vi "HFRR ADV v011 new software.vi"() -> ()   [LabVIEW 2025] (continued)
            n938 = local write "LIVE FEED MIN TEMP"(w1292) -> ()
            n939 = call "CAMERA LIVE FEED FGV.vi"("Enum - Menu"=CAMERA_LIVE_FEED_ENUM."CAMERA MINIMIZE") -> ()  [unwired: 9 in, 2 out]
          }
        }
        n940 = case shown="True" w1284 {
          selector: w1284 -> [_ w1290]
          frame False {
          }
          frame True {
            n941 = Not(x=w1290) -> (.not. x?=w1289:bool)
            n942 = local write "CAMERA ROI MIN TEMP"(w1289) -> ()
            n943 = call "IMAGE ANALYSIS.vi"("Enum"=POST_ANALYSIS_ENUM."MINIMIZE UI") -> ()  [unwired: 9 in, 2 out]
          }
        }
        n944 = local write "CAMERA ROI MAX TEMP"(TRUE ("CAMERA ROI MAX TEMP")) -> ()
      }
      frame "About" {
        n945 = local read "LIVE FEED MIN TEMP"() -> (w1296:bool)
        n946 = local write "LIVE FEED MAX TEMP"(TRUE ("LIVE FEED MAX TEMP")) -> ()
        n947 = local read "CAMERA ROI MIN TEMP"() -> (w1295:bool)
        n948 = case shown="True" w1296 {
          selector: w1296 -> [_ w1303]
          frame False {
          }
          frame True {
            n949 = Not(x=w1303) -> (.not. x?=w1302:bool)
            n950 = local write "LIVE FEED MIN TEMP"(w1302) -> ()
            n951 = call "CAMERA LIVE FEED FGV.vi"("Enum - Menu"=CAMERA_LIVE_FEED_ENUM."CAMERA MINIMIZE") -> ()  [unwired: 9 in, 2 out]
          }
        }
        n952 = case shown="True" w1295 {
          selector: w1295 -> [_ w1300]
          frame False {
          }
          frame True {
            n953 = Not(x=w1300) -> (.not. x?=w1299:bool)
            n954 = local write "CAMERA ROI MIN TEMP"(w1299) -> ()
            n955 = call "IMAGE ANALYSIS.vi"("Enum"=POST_ANALYSIS_ENUM."MINIMIZE UI") -> ()  [unwired: 9 in, 2 out]
          }
        }
        n956 = local write "CAMERA ROI MAX TEMP"(TRUE ("CAMERA ROI MIN TEMP")) -> ()
      }
      frame "Advance" {
        n957 = local read "LIVE FEED MIN TEMP"() -> (w1306:bool)
        n958 = local write "LIVE FEED MAX TEMP"(TRUE ("LIVE FEED MAX TEMP")) -> ()
        n959 = local read "CAMERA ROI MIN TEMP"() -> (w1304:bool)
        n960 = case shown="True" w1306 {
          selector: w1306 -> [_ w1313]
          frame False {
          }
          frame True {
            n961 = Not(x=w1313) -> (.not. x?=w1312:bool)
            n962 = local write "LIVE FEED MIN TEMP"(w1312) -> ()
            n963 = call "CAMERA LIVE FEED FGV.vi"("Enum - Menu"=CAMERA_LIVE_FEED_ENUM."CAMERA MINIMIZE") -> ()  [unwired: 9 in, 2 out]
          }
        }
        n964 = local write "CAMERA ROI MAX TEMP"(TRUE ("CAMERA ROI MAX TEMP")) -> ()
        n965 = case shown="True" w1304 {
          selector: w1304 -> [_ w1310]
          frame False {
          }
          frame True {
            n966 = Not(x=w1310) -> (.not. x?=w1309:bool)
            n967 = local write "CAMERA ROI MIN TEMP"(w1309) -> ()
            n968 = call "IMAGE ANALYSIS.vi"("Enum"=POST_ANALYSIS_ENUM."MINIMIZE UI") -> ()  [unwired: 9 in, 2 out]
          }
        }
      }
      frame "Mooha" {
        n969 = local read "LIVE FEED MIN TEMP"() -> (w1316:bool)
        n970 = local write "LIVE FEED MAX TEMP"(TRUE ("LIVE FEED MAX TEMP")) -> ()
        n971 = local read "CAMERA ROI MIN TEMP"() -> (w1314:bool)
        n972 = case shown="True" w1316 {
          selector: w1316 -> [_ w1323]
          frame False {
          }
          frame True {
            n973 = Not(x=w1323) -> (.not. x?=w1322:bool)
            n974 = local write "LIVE FEED MIN TEMP"(w1322) -> ()
            n975 = call "CAMERA LIVE FEED FGV.vi"("Enum - Menu"=CAMERA_LIVE_FEED_ENUM."CAMERA MINIMIZE") -> ()  [unwired: 9 in, 2 out]
          }
        }
        n976 = local write "CAMERA ROI MAX TEMP"(TRUE ("CAMERA ROI MAX TEMP")) -> ()
        n977 = case shown="True" w1314 {
          selector: w1314 -> [_ w1320]
          frame False {
          }
          frame True {
            n978 = Not(x=w1320) -> (.not. x?=w1319:bool)
            n979 = local write "CAMERA ROI MIN TEMP"(w1319) -> ()
            n980 = call "IMAGE ANALYSIS.vi"("Enum"=POST_ANALYSIS_ENUM."MINIMIZE UI") -> ()  [unwired: 9 in, 2 out]
          }
        }
      }
    }
    n981 = local read "Auto Start Test"() -> (w1060:bool)
    n982 = case shown="True" "sign in temp" {
      frame False {
      }
      frame True {
        w1096 = 1 ("y")
        n983 = local read "USERNAME"() -> (w1102:string)
        n984 = local read "USER ID"() -> (w1099:string)
        n985 = call <vilib>:"Trim Whitespace.vi"("string"=w1102) -> ("trimmed string"=w1101:string)  [unwired: 1 in]
        n986 = call <vilib>:"Trim Whitespace.vi"("string"=w1099) -> ("trimmed string"=w1100:string)  [unwired: 1 in]
        n987 = String Length(string=w1101) -> (length=w1098:i32)
        n988 = String Length(string=w1100) -> (length=w1097:i32)
        n989 = Greater?(x=w1098, y=w1096) -> (0:w1095:bool)
        n990 = Greater?(x=w1097, y=w1096) -> (0:w1094:bool)
        n991 = And(x=w1095, y=w1094) -> (x .and. y?=w1093:bool)
        n992 = case shown="True" w1093 {
          frame False {
            n993 = property on="Sign In" class="Bool (strict)"("DisabledEnum"=T17."Disabled" ("Disabled")) -> ()  [unwired: 2 in, 2 out]
          }
          frame True {
            n994 = property on="Sign In" class="Bool (strict)"("DisabledEnum"=T17."Enabled" ("Disabled")) -> ()  [unwired: 2 in, 2 out]
          }
        }
      }
    }
    n995 = local read "Air Temperature"() -> (w1077:bool)
    n996 = local read "Coefficient Of Friction"() -> (w1078:bool)
    n997 = case shown="False" w1060 {
      frame False {
        n998 = local read "Auto stop temp"() -> (w1090:bool)
        n999 = case shown="True" w1090 {
          frame False {
          }
          frame True {
            n1000 = local write "Auto Start Temp"(FALSE ("Auto Start Temp")) -> ()
          }
        }
      }
      frame True {
        "Auto stop temp" <- TRUE ("Auto stop temp")
      }
    }
    n1001 = local read "Humidity"() -> (w1076:bool)
    n1002 = case shown="\"HOME\"" w1087 {
      frame "HOME" {
        n1003 = local write "main tab sub"(enum32{"Page 1", "Page 2"}."Page 1" ("main tab sub")) -> ()
      }
      frame Default {
        n1004 = local write "main tab sub"(enum32{"Page 1", "Page 2"}."Page 2" ("main tab sub")) -> ()
      }
    }
    n1005 = case shown="True" w1086 {
      selector: w1086 -> [_ w1437]
      frame False {
      }
      frame True {
        n1006 = Not(x=w1437) -> (.not. x?=w1436:bool)
        n1007 = local write "Sign In"(w1436) -> ()
        n1008 = local write "Main Dashboard Buttons"(T23."Test Setup" ("Main Dashboard Buttons")) -> ()
      }
    }
    n1009 = case shown="\"Numeric Display\", Default" "Num/Graph" {
      frame "Numeric Display", Default {
        n1010 = property on="Single/Multiple" class="RadioBtnsControl (strict)"("Visible"=FALSE) -> ()  [unwired: 2 in, 2 out]
        n1011 = property on="Single - Graph" class="Ring (strict)"("Visible"=FALSE) -> ()  [unwired: 2 in, 2 out]
        n1012 = local write "Main Tab Display"(T4."Dashboard 1" ("Main Tab Display")) -> ()
      }
      frame "Graph Display" {
        n1013 = property on="Single/Multiple" class="RadioBtnsControl (strict)"("Visible"=TRUE) -> ()  [unwired: 2 in, 2 out]
        n1014 = case shown="\"Multiple\"" "Single/Multiple" {
          frame "Single ", Default {
            n1015 = property on="Single - Graph" class="Ring (strict)"("Visible"=TRUE) -> ()  [unwired: 2 in, 2 out]
            n1016 = local write "Main Tab Display"(T4."Dashboard 3" ("Main Tab Display")) -> ()
          }
          frame "Multiple" {
            n1017 = property on="Single - Graph" class="Ring (strict)"("Visible"=FALSE) -> ()  [unwired: 2 in, 2 out]
            n1018 = local write "Main Tab Display"(T4."Dashboard 2" ("Main Tab Display")) -> ()
          }
        }
      }
    }
    n1019 = local read "Stroke"() -> (w1075:bool)
    n1020 = local read "USERNAME"() -> (w1081:string)
    n1021 = local read "USER ID"() -> (w1080:string)
    n1022 = case shown="True" w1078 {
      selector: w1078 -> [_ w1363]
      frame False {
      }
      frame True {
        n1023 = Not(x=w1363) -> (.not. x?=w1362:bool)
        n1024 = local write "Coefficient Of Friction"(w1362) -> ()
        n1025 = local write "Tab Control 2"(T6."Coefficient Of Friction" ("Tab Control 2")) -> ()
      }
    }
    n1026 = case shown="True" w1077 {
      selector: w1077 -> [_ w1360]
      frame False {
      }
      frame True {
        n1027 = Not(x=w1360) -> (.not. x?=w1358:bool)
        n1028 = local write "Air Temperature"(w1358) -> ()
        n1029 = local write "Tab Control 2"(T6."Air Temperature" ("Tab Control 2")) -> ()
      }
    }
    n1030 = local write "Operator ID"(w1080) -> ()
    n1031 = case shown="True" w1075 {
      selector: w1075 -> [_ w1354]
      frame False {
      }
      frame True {
        n1032 = Not(x=w1354) -> (.not. x?=w1352:bool)
        n1033 = local write "Stroke"(w1352) -> ()
        n1034 = local write "Tab Control 2"(T6."Stroke" ("Tab Control 2")) -> ()
      }
    }
    n1035 = local write "tested by"(w1081) -> ()
    n1036 = case shown="True" w1076 {
      selector: w1076 -> [_ w1357]
      frame False {
      }
      frame True {
        n1037 = Not(x=w1357) -> (.not. x?=w1355:bool)
        n1038 = local write "Humidity"(w1355) -> ()
        n1039 = local write "Tab Control 2"(T6."Humidity" ("Tab Control 2")) -> ()
      }
    }
    n1040 = case shown="\"Calibration\"" "Main Dashboard Buttons" {
      tunnel: [T2."HOME" ("Main Tab") T2."Test Setup" ("Main Tab") T2."Acquire" ("Main Tab") T2."Adv Scar" ("Main Tab") T2."Adv Scar Report" ("Main Tab") T2."Compare Files" ("Main Tab") T2."Calibration" ("Main Tab") T2."About" ("Main Tab") T2."Advance" ("Main Tab")] -> w1059
      frame "Home", Default {
      }
      frame "Test Setup" {
      }
      frame "Dashboard" {
      }
      frame "Imaging" {
      }
      frame "Report" {
      }
      frame "Analysis" {
      }
      frame "Calibration" {
      }
      frame "About" {
      }
      frame "Advance" {
      }
    }
    n1041 = Wait (ms)(milliseconds to wait=u32 100) -> ()  [unwired: 1 out]
    n1042 = local read "Main Tab Display"() -> (w1079:T4)
    n1043 = local write "Main Tab"(w1059) -> ()
    n1044 = case shown="\"Dashboard 3\"" w1079 {
      frame "Dashboard 1", Default {
        n1045 = property on="Reset Graph" class="Bool (strict)"("Visible"=FALSE) -> ()  [unwired: 2 in, 2 out]
      }
      frame "Dashboard 2" {
        n1046 = property on="Reset Graph" class="Bool (strict)"("Visible"=TRUE) -> ()  [unwired: 2 in, 2 out]
      }
      frame "Dashboard 3" {
        n1047 = property on="Reset Graph" class="Bool (strict)"("Visible"=TRUE) -> ()  [unwired: 2 in, 2 out]
      }
    }
    n1048 = local read "SCAR MEASURMENT"() -> (w1067:enum32{"Auto Scar", "Manual Scar"})
    n1049 = local read "Humidity"() -> (w1082:bool)
    n1050 = local read "Cap Live Image"() -> (w1064:bool)
    n1051 = local read "Sample Temperature"() -> (w1074:bool)
    n1052 = local read "Air Temp vs Humidity"() -> (w1072:bool)
    n1053 = local read "Frequency"() -> (w1073:bool)
    n1054 = case shown="True" w1082 {
      frame False {
        n1055 = local write "Humidity On Command"(TRUE ("Humidity On Command")) -> ()
        n1056 = case shown="True" "Humidity Off Command" {
          selector: "Humidity Off Command" -> [_ w1370]
          frame False {
          }
          frame True {
            n1057 = stacked-sequence {
              frame #0 {
                n1058 = local read "WriteHumidity"() -> (w1372:string[])
                n1059 = Insert Into Array(array=w1372, new element="R;1" ("new element/subarray")) -> (w1373:string[])  [unwired: 1 in]
                n1060 = local write "WriteHumidity"(w1373) -> ()
              }
              frame #1 {
                n1061 = Wait (ms)(milliseconds to wait=u32 2000) -> ()  [unwired: 1 out]
              }
              frame #2 {
                n1062 = local read "EVENT LOG"() -> (w1379:string)
                n1063 = local read "WriteHumidity"() -> (w1376:string[])
                n1064 = call "Event Log.vi"("Content"="Humidity Control Off" ("string"), "EVENT LOG"=w1379) -> ("EVENT LOG"=w1380:string)  [unwired: 8 in, 1 out]
                n1065 = local write "EVENT LOG"(w1380) -> ()
                n1066 = Insert Into Array(array=w1376, new element="R;1" ("new element/subarray")) -> (w1377:string[])  [unwired: 1 in]
                n1067 = local write "WriteHumidity"(w1377) -> ()
              }
            }
            n1068 = Not(x=w1370) -> (.not. x?=w1369:bool)
            n1069 = local write "Humidity Off Command"(w1369) -> ()
          }
        }
      }
      frame True {
        n1070 = local write "Humidity Off Command"(TRUE ("Humidity Off Command")) -> ()
        n1071 = case shown="True" "Humidity On Command" {
          selector: "Humidity On Command" -> [_ w1384]
          frame False {
          }
          frame True {
            n1072 = stacked-sequence {
              frame #0 {
                n1073 = local read "Set Rh"() -> (w1390:dbl)
                n1074 = Number To Fractional String(number=w1390, precision (6)=i16 2) -> (F-format string=w1391:string)  [unwired: 2 in]
                n1075 = local read "WriteHumidity"() -> (w1388:string[])
                n1076 = Concatenate Strings("M;" ("new element/subarray"), w1391) -> (w1389:string)
                n1077 = Insert Into Array(array=w1388, new element=w1389) -> (w1387:string[])  [unwired: 1 in]
                n1078 = local write "WriteHumidity"(w1387) -> ()
              }
              frame #1 {
                n1079 = Wait (ms)(milliseconds to wait=u32 2000) -> ()  [unwired: 1 out]
              }
              frame #2 {
                n1080 = local read "Set Rh"() -> (w1398:dbl)
                n1081 = Number To Fractional String(number=w1398, precision (6)=i16 2) -> (F-format string=w1399:string)  [unwired: 2 in]
                n1082 = local read "WriteHumidity"() -> (w1396:string[])
                n1083 = Concatenate Strings("M;" ("new element/subarray"), w1399) -> (w1397:string)
                n1084 = Insert Into Array(array=w1396, new element=w1397) -> (w1395:string[])  [unwired: 1 in]
                n1085 = local write "WriteHumidity"(w1395) -> ()
              }
              frame #3 {
                n1086 = Wait (ms)(milliseconds to wait=u32 1500) -> ()  [unwired: 1 out]
              }
              frame #4 {
                (unwired) "% RH" ("string")
                (unwired) i16 2 ("precision (6)")
                (unwired) "M;" ("new element/subarray")
                n1087 = local read "Set Rh"() -> (w1406:dbl)
                n1088 = Number To Fractional String(number=w1406, precision (6)=i16 2) -> (F-format string=w1403:string)  [unwired: 2 in]
                n1089 = local read "WriteHumidity"() -> (w1408:string[])
                n1090 = Concatenate Strings("M;" ("new element/subarray"), w1403) -> (w1407:string)
                n1091 = Concatenate Strings("Humidity Set to : " ("string"), w1403, "% RH" ("string")) -> (w1401:string)
                n1092 = Insert Into Array(array=w1408, new element=w1407) -> (w1409:string[])  [unwired: 1 in]
                n1093 = disable-structure shown="Enabled" {
                  frame Enabled {
                    n1094 = local read "EVENT LOG"() -> (w1412:string)
                    n1095 = call "Event Log.vi"("Content"="Humidity Control On", "EVENT LOG"=w1412) -> ("EVENT LOG"=w1413:string)  [unwired: 8 in, 1 out]
                    n1096 = local write "EVENT LOG"(w1413) -> ()
                  }
                  frame Disabled {
                  }
                }
                n1097 = disable-structure shown="Enabled" {
                  disable-tunnel: w1401 -> [_ _]
                  frame Enabled {
                    n1098 = local read "EVENT LOG"() -> (w1415:string)
                    n1099 = call "Event Log.vi"("Content"="Humidity Control On", "EVENT LOG"=w1415) -> ("EVENT LOG"=w1416:string)  [unwired: 8 in, 1 out]
                    n1100 = local write "EVENT LOG"(w1416) -> ()
                  }
                  frame Disabled {
                  }
                }
                n1101 = local write "WriteHumidity"(w1409) -> ()
              }
            }
            n1102 = Not(x=w1384) -> (.not. x?=w1383:bool)
            n1103 = local write "Humidity On Command"(w1383) -> ()
          }
        }
      }
    }
    n1104 = Equal?(x=w1067, y=enum32{"Auto Scar", "Manual Scar"}."Auto Scar" ("SCAR MEASURMENT")) -> (x = y?=w1063:bool)
    n1105 = local read "TEST STANDARD"() -> (w1070:T3)
    n1106 = And(x=w1064, y=w1063) -> (x .and. y?=w1065:bool)
    n1107 = case shown="True" w1065 {
      selector: w1065 -> [_ w1169]
      tunnel: errorcluster {"status"=FALSE, "code"=0, "source"=""} ("error in (no error) 3") -> [_ w1170]
      frame False {
      }
      frame True {
        n1108 = stacked-sequence {
          tunnel: w1170 -> [_ _ _ _ _ _ _ w1218]
          tunnel: w1169 -> [_ _ _ _ _ w1199 _ _]
          frame #0 {
            n1109 = call "CAMERA LIVE FEED FGV.vi"("Enum - Menu"=CAMERA_LIVE_FEED_ENUM."CAMERA MINIMIZE") -> ()  [unwired: 9 in, 2 out]
          }
          frame #1 {
            n1110 = property on="Auto Scar Check  2" class="Clust (strict)"("Visible"=TRUE) -> ()  [unwired: 2 in, 2 out]
          }
          frame #2 {
            n1111 = String To Path(string="C:\\LAB-IQ\\Image Calibrate v01.dcf") -> (path=w1175:path)
            n1112 = Open/Create/Replace File ("Open File")(file path (use dialog)=w1175) -> (refnum out=w1176:refnum<file>)  [unwired: 5 in, 2 out]
            n1113 = for {
              N: 4 -> [_]
              tunnel: w1176 -> [w1182]
              i -> [w1178]
              n1114 = Read from Text File ("Read File")(file (use dialog)=w1182) -> (text=w1183:string)  [unwired: 3 in, 3 out]
              n1115 = String Subset(string=w1183, offset (0)=6, length (rest)=10 ("length (rest)")) -> (substring=w1179:string)
              n1116 = Fract/Exp String To Number(string=w1179) -> (number=w1177:dbl)  [unwired: 3 in, 1 out]
              n1117 = case shown="0" w1178 {
                tunnel: w1177 -> [w1184 w1185 _ w1186 _]
                frame 0 {
                  "5x Gain" <- w1184
                }
                frame 1 {
                  "10x Gain" <- w1185
                }
                frame 2 {
                }
                frame 3 {
                  "100x gain" <- w1186
                }
                frame 4, Default {
                }
              }
            }
          }
          frame #3 {
            n1118 = local read "FILE 3"() -> (w1192:string)
            n1119 = call <vilib>:"Trim Whitespace.vi"("string"="C:\\LAB-IQ\\images\\") -> ("trimmed string"=w1194:string)  [unwired: 1 in]
            n1120 = String To Path(string=w1194) -> (path=w1193:path)
            n1121 = Concatenate Strings(w1192, ".png" ("string")) -> (w1191:string)
            n1122 = Build Path(base path=w1193, name or relative path=w1191) -> (appended path=w1189:path)
            "Image path" <- w1189
            n1123 = Path To String(path=w1189) -> (string=w1188:string)
            n1124 = call "CAMERA LIVE FEED FGV.vi"("Enum - Menu"=CAMERA_LIVE_FEED_ENUM."CAMERA SAVE", "Image Path"=w1188) -> ()  [unwired: 8 in, 2 out]
          }
          frame #4 {
            n1125 = One Button Dialog(message="Image saved successfully") -> ()  [unwired: 1 in, 1 out]
          }
          frame #5 {
            n1126 = local read "TEST STANDARD"() -> (w1198:T3)
            n1127 = local read "Magnification len live scar"() -> (w1210:string)
            n1128 = Not(x=w1199) -> (.not. x?=w1200:bool)
            n1129 = local write "Cap Live Image"(w1200) -> ()
            n1130 = case shown="\"ISO 12156\"" w1198 {
              tunnel: ["ASTM D6079" "ISO 12156"] -> w1197
              frame "ASTM D6079", Default {
              }
              frame "ISO 12156" {
              }
            }
            n1131 = case shown="\"5x\", Default" w1210 {
              tunnel: [w1213 w1214] -> w1209
              frame "5x", Default {
                n1132 = local read "5x Gain"() -> (w1213:dbl)
              }
              frame "10x" {
                # "5x"
                n1133 = local read "10x Gain"() -> (w1214:dbl)
              }
            }
            n1134 = local read "Image path"() -> (w1208:path)
            n1135 = local read "FILE 3"() -> (w1201:string)
            n1136 = call "EDGE DETCTION.vi"("GAIN VALUE"=w1209, "Image Path"=w1208) -> ("error out"=w1207:errorcluster, "return value"=w1206:cluster{string, string, dbl, dbl, dbl})  [unwired: 8 in]
            n1137 = Bundle By Name(cluster=T24 {"File Name"="", "Test Method"="", "Operator"="", "Fuel Description"="", "Date and time"=""} ("Main Ref"), "File Name"=w1201, "Test Method"=w1197) -> (w1202:T24)
            n1138 = call "duf file read.vi"("error in (no error)"=w1207, "Main Ref"=w1202) -> ("error out"=w1205:errorcluster, "Main Ref 2"=w1203:T24)  [unwired: 8 in]
            n1139 = call "EDGE DETECTION REPORT.vi"("error in (no error)"=w1205, "return value 2"=w1206, "Main Ref"=w1203) -> ()  [unwired: 8 in, 1 out]
          }
          frame #6 {
            n1140 = property on="Auto Scar Check  2" class="Clust (strict)"("Visible"=FALSE) -> ()  [unwired: 2 in, 2 out]
          }
          frame #7 {
            n1141 = call "CAMERA LIVE FEED FGV.vi"("Enum - Menu"=CAMERA_LIVE_FEED_ENUM."CAMERA MINIMIZE", "error in (no error)"=w1218) -> ()  [unwired: 8 in, 2 out]
            n1142 = local write "Main Dashboard Buttons"(T1."Home" ("Main Dashboard Buttons")) -> ()
            n1143 = local write "Main Tab"(T2."HOME" ("Main Tab")) -> ()
          }
        }
      }
    }
    n1144 = local read "Heater Button"() -> (w1071:bool)
    n1145 = case shown="True" w1073 {
      selector: w1073 -> [_ w1348]
      frame False {
      }
      frame True {
        n1146 = Not(x=w1348) -> (.not. x?=w1346:bool)
        n1147 = local write "Frequency"(w1346) -> ()
        n1148 = local write "Tab Control 2"(T6."Frequency" ("Tab Control 2")) -> ()
      }
    }
    n1149 = case shown="True" w1072 {
      selector: w1072 -> [_ w1345]
      frame False {
      }
      frame True {
        n1150 = Not(x=w1345) -> (.not. x?=w1343:bool)
        n1151 = local write "Air Temp vs Humidity"(w1343) -> ()
        n1152 = local write "Tab Control 2"(T6."Air Temp vs Rh" ("Tab Control 2")) -> ()
      }
    }
    n1153 = case shown="True" w1074 {
      selector: w1074 -> [_ w1351]
      frame False {
      }
      frame True {
        n1154 = Not(x=w1351) -> (.not. x?=w1349:bool)
        n1155 = local write "Sample Temperature"(w1349) -> ()
        n1156 = local write "Tab Control 2"(T6."Sample Temperature" ("Tab Control 2")) -> ()
      }
    }
    n1157 = case shown="\"Custom\"" w1070 {
      frame "ASTM D6079", Default {
        w1324 = "ASTM D6079 TEST CONDITIONS" ("Standard 2")
        n1158 = local write "Standard 2"(w1324) -> ()
        n1159 = local write "Standard"(w1324) -> ()
      }
      frame "ISO 12156" {
        w1325 = "ISO 12156 TEST CONDITIONS" ("Standard 2")
        n1160 = local write "Standard 2"(w1325) -> ()
        n1161 = local write "Standard"(w1325) -> ()
      }
      frame "CEC F-096-A-06" {
        w1326 = "CEC F-096-A-06 TEST CONDITIONS" ("Standard 2")
        n1162 = local write "Standard 2"(w1326) -> ()
        n1163 = local write "Standard"(w1326) -> ()
      }
      frame "Custom" {
        w1327 = "CUSTOM TEST CONDITIONS" ("Standard 2")
        n1164 = local write "Standard 2"(w1327) -> ()
        n1165 = local write "Standard"(w1327) -> ()
      }
    }
    n1166 = case shown="True" w1071 {
      frame False {
        n1167 = local write "Temperature On Command"(TRUE ("Temperature On Command")) -> ()
        n1168 = case shown="True" "Temperature Off Command" {
          selector: "Temperature Off Command" -> [_ w1331]
          frame False {
          }
          frame True {
            n1169 = Not(x=w1331) -> (.not. x?=w1330:bool)
            n1170 = local read "EVENT LOG"() -> (w1334:string)
            n1171 = local write "Temperature Off Command"(w1330) -> ()
            n1172 = call "Event Log.vi"("Content"="Heater Off", "EVENT LOG"=w1334) -> ("EVENT LOG"=w1333:string)  [unwired: 8 in, 1 out]
            n1173 = local write "EVENT LOG"(w1333) -> ()
          }
        }
      }
      frame True {
        n1174 = local write "Temperature Off Command"(TRUE ("Temperature Off Command")) -> ()
        n1175 = case shown="True" "Temperature On Command" {
          selector: "Temperature On Command" -> [_ w1338]
          frame False {
          }
          frame True {
            n1176 = Not(x=w1338) -> (.not. x?=w1337:bool)
            n1177 = local write "Temperature On Command"(w1337) -> ()
            n1178 = disable-structure shown="Enabled" {
              disable-tunnel: "Heater On" -> [w1340 _]
              frame Enabled {
                n1179 = local read "EVENT LOG"() -> (w1341:string)
                n1180 = call "Event Log.vi"("Content"=w1340, "EVENT LOG"=w1341) -> ("EVENT LOG"=w1342:string)  [unwired: 8 in, 1 out]
                n1181 = local write "EVENT LOG"(w1342) -> ()
              }
              frame Disabled {
              }
            }
          }
        }
      }
    }
    n1182 = local read "Main Tab"() -> (w1062:T2)
    n1183 = case shown="\"About\"" w1062 {
      frame "HOME", Default {
        w1105 = T17."Enabled" ("Disabled")
        n1184 = local read "Service Password enable"() -> (w1107:bool)
        n1185 = property on="Imaging" class="Bool (strict)"("DisabledEnum"=w1105) -> ()  [unwired: 2 in, 2 out]
        n1186 = property on="Dashboard" class="Bool (strict)"("DisabledEnum"=w1105) -> ()  [unwired: 2 in, 2 out]
        n1187 = property on="Test Setup" class="Bool (strict)"("DisabledEnum"=w1105) -> ()  [unwired: 2 in, 2 out]
        n1188 = property on="Analysis" class="Bool (strict)"("DisabledEnum"=w1105) -> ()  [unwired: 2 in, 2 out]
        n1189 = property on="Home" class="Bool (strict)"("DisabledEnum"=w1105) -> ()  [unwired: 2 in, 2 out]
        n1190 = property on="Report" class="Bool (strict)"("DisabledEnum"=w1105) -> ()  [unwired: 2 in, 2 out]
        n1191 = property on="Main Dashboard Buttons" class="RadioBtnsControl (strict)"("DisabledEnum"=w1105) -> ()  [unwired: 2 in, 2 out]
        n1192 = property on="Calibration" class="Bool (strict)"("DisabledEnum"=w1105) -> ()  [unwired: 2 in, 2 out]
        n1193 = case shown="True" w1107 {
          tunnel: [T17."Disabled" ("Disabled") T17."Enabled" ("Disabled")] -> w1106
          frame False {
          }
          frame True {
          }
        }
        n1194 = property on="About" class="Bool (strict)"("DisabledEnum"=w1106) -> ()  [unwired: 2 in, 2 out]
      }
      frame "Test Setup" {
        w1112 = T17."Enabled" ("Disabled")
        n1195 = local read "Service Password enable"() -> (w1111:bool)
        n1196 = property on="Dashboard" class="Bool (strict)"("DisabledEnum"=T17."Disabled" ("Disabled")) -> ()  [unwired: 2 in, 2 out]
        n1197 = property on="Imaging" class="Bool (strict)"("DisabledEnum"=w1112) -> ()  [unwired: 2 in, 2 out]
        n1198 = property on="Analysis" class="Bool (strict)"("DisabledEnum"=w1112) -> ()  [unwired: 2 in, 2 out]
        n1199 = property on="Home" class="Bool (strict)"("DisabledEnum"=w1112) -> ()  [unwired: 2 in, 2 out]
        n1200 = property on="Report" class="Bool (strict)"("DisabledEnum"=w1112) -> ()  [unwired: 2 in, 2 out]
        n1201 = property on="Test Setup" class="Bool (strict)"("DisabledEnum"=w1112) -> ()  [unwired: 2 in, 2 out]
        n1202 = case shown="True" w1111 {
          tunnel: [T17."Disabled" ("Disabled") T17."Enabled" ("Disabled")] -> w1110
          frame False {
          }
          frame True {
          }
        }
        n1203 = property on="About" class="Bool (strict)"("DisabledEnum"=w1110) -> ()  [unwired: 2 in, 2 out]
      }
      frame "Adv Scar" {
        w1119 = T17."Enabled" ("Disabled")
        n1204 = property on="Dashboard" class="Bool (strict)"("DisabledEnum"=T17."Disabled" ("Disabled")) -> ()  [unwired: 2 in, 2 out]
        n1205 = property on="Imaging" class="Bool (strict)"("DisabledEnum"=w1119) -> ()  [unwired: 2 in, 2 out]
        n1206 = property on="Analysis" class="Bool (strict)"("DisabledEnum"=w1119) -> ()  [unwired: 2 in, 2 out]
        n1207 = property on="Home" class="Bool (strict)"("DisabledEnum"=w1119) -> ()  [unwired: 2 in, 2 out]
        n1208 = property on="Report" class="Bool (strict)"("DisabledEnum"=w1119) -> ()  [unwired: 2 in, 2 out]
        n1209 = property on="Test Setup" class="Bool (strict)"("DisabledEnum"=w1119) -> ()  [unwired: 2 in, 2 out]
        n1210 = local read "Service Password enable"() -> (w1117:bool)
        n1211 = case shown="True" w1117 {
          tunnel: [T17."Disabled" ("Disabled") T17."Enabled" ("Disabled")] -> w1116
          frame False {
          }
          frame True {
          }
        }
        n1212 = property on="About" class="Bool (strict)"("DisabledEnum"=w1116) -> ()  [unwired: 2 in, 2 out]
      }
      frame "Calibration" {
        w1122 = T17."Enabled" ("Disabled")
        n1213 = property on="Dashboard" class="Bool (strict)"("DisabledEnum"=T17."Disabled" ("Disabled")) -> ()  [unwired: 2 in, 2 out]
        n1214 = property on="Imaging" class="Bool (strict)"("DisabledEnum"=w1122) -> ()  [unwired: 2 in, 2 out]
        n1215 = property on="Analysis" class="Bool (strict)"("DisabledEnum"=w1122) -> ()  [unwired: 2 in, 2 out]
        n1216 = property on="Home" class="Bool (strict)"("DisabledEnum"=w1122) -> ()  [unwired: 2 in, 2 out]
        n1217 = property on="Report" class="Bool (strict)"("DisabledEnum"=w1122) -> ()  [unwired: 2 in, 2 out]
        n1218 = property on="Test Setup" class="Bool (strict)"("DisabledEnum"=w1122) -> ()  [unwired: 2 in, 2 out]
        n1219 = local read "Service Password enable"() -> (w1124:bool)
        n1220 = property on="Calibration" class="Bool (strict)"("DisabledEnum"=w1122) -> ()  [unwired: 2 in, 2 out]
        n1221 = case shown="True" w1124 {
          tunnel: [T17."Disabled" ("Disabled") T17."Enabled" ("Disabled")] -> w1123
          frame False {
          }
          frame True {
          }
        }
        n1222 = property on="About" class="Bool (strict)"("DisabledEnum"=w1123) -> ()  [unwired: 2 in, 2 out]
      }
      frame "Adv Scar Report" {
        w1130 = T17."Enabled" ("Disabled")
        n1223 = property on="Dashboard" class="Bool (strict)"("DisabledEnum"=T17."Disabled" ("Disabled")) -> ()  [unwired: 2 in, 2 out]
        n1224 = property on="Imaging" class="Bool (strict)"("DisabledEnum"=w1130) -> ()  [unwired: 2 in, 2 out]
        n1225 = property on="Analysis" class="Bool (strict)"("DisabledEnum"=w1130) -> ()  [unwired: 2 in, 2 out]
        n1226 = property on="Home" class="Bool (strict)"("DisabledEnum"=w1130) -> ()  [unwired: 2 in, 2 out]
        n1227 = property on="Report" class="Bool (strict)"("DisabledEnum"=w1130) -> ()  [unwired: 2 in, 2 out]
        n1228 = property on="Test Setup" class="Bool (strict)"("DisabledEnum"=w1130) -> ()  [unwired: 2 in, 2 out]
        n1229 = local read "Service Password enable"() -> (w1129:bool)
        n1230 = case shown="True" w1129 {
          tunnel: [T17."Disabled" ("Disabled") T17."Enabled" ("Disabled")] -> w1128
          frame False {
          }
          frame True {
          }
        }
        n1231 = property on="About" class="Bool (strict)"("DisabledEnum"=w1128) -> ()  [unwired: 2 in, 2 out]
      }
      frame "Compare Files" {
        w1136 = T17."Enabled" ("Disabled")
        n1232 = local read "Service Password enable"() -> (w1135:bool)
        n1233 = property on="Dashboard" class="Bool (strict)"("DisabledEnum"=T17."Disabled" ("Disabled")) -> ()  [unwired: 2 in, 2 out]
        n1234 = property on="Imaging" class="Bool (strict)"("DisabledEnum"=w1136) -> ()  [unwired: 2 in, 2 out]
        n1235 = property on="Analysis" class="Bool (strict)"("DisabledEnum"=w1136) -> ()  [unwired: 2 in, 2 out]
        n1236 = property on="Home" class="Bool (strict)"("DisabledEnum"=w1136) -> ()  [unwired: 2 in, 2 out]
        n1237 = property on="Report" class="Bool (strict)"("DisabledEnum"=w1136) -> ()  [unwired: 2 in, 2 out]
        n1238 = property on="Test Setup" class="Bool (strict)"("DisabledEnum"=w1136) -> ()  [unwired: 2 in, 2 out]
        n1239 = case shown="True" w1135 {
          tunnel: [T17."Disabled" ("Disabled") T17."Enabled" ("Disabled")] -> w1134
          frame False {
          }
          frame True {
          }
        }
        n1240 = property on="About" class="Bool (strict)"("DisabledEnum"=w1134) -> ()  [unwired: 2 in, 2 out]
      }
      frame "Acquire" {
        n1241 = local read "Service Password enable"() -> (w1141:bool)
        n1242 = property on="Test Setup" class="Bool (strict)"("DisabledEnum"=T17."Disabled" ("Disabled")) -> ()  [unwired: 2 in, 2 out]
        n1243 = local read "Auto Start Test"() -> (w1143:bool)
        n1244 = local read "RUN"() -> (w1145:bool)
        n1245 = case shown="True" w1141 {
          tunnel: [T17."Disabled" ("Disabled") T17."Enabled" ("Disabled")] -> w1142
          frame False {
          }
          frame True {
          }
        }
        n1246 = Or(x=w1145, y=w1143) -> (x .or. y?=w1144:bool)
        n1247 = case shown="True" w1144 {
          tunnel: [T17."Enabled" ("Disabled") T17."Disabled" ("Disabled")] -> w1140
          frame False {
          }
          frame True {
          }
        }
        n1248 = property on="About" class="Bool (strict)"("DisabledEnum"=w1142) -> ()  [unwired: 2 in, 2 out]
        n1249 = property on="Imaging" class="Bool (strict)"("DisabledEnum"=w1140) -> ()  [unwired: 2 in, 2 out]
        n1250 = property on="Dashboard" class="Bool (strict)"("DisabledEnum"=w1140) -> ()  [unwired: 2 in, 2 out]
        n1251 = property on="Analysis" class="Bool (strict)"("DisabledEnum"=w1140) -> ()  [unwired: 2 in, 2 out]
        n1252 = property on="Home" class="Bool (strict)"("DisabledEnum"=w1140) -> ()  [unwired: 2 in, 2 out]
        n1253 = property on="Report" class="Bool (strict)"("DisabledEnum"=w1140) -> ()  [unwired: 2 in, 2 out]
        n1254 = property on="Calibration" class="Bool (strict)"("DisabledEnum"=w1140) -> ()  [unwired: 2 in, 2 out]
      }
      frame "About" {
        n1255 = local read "FILE"() -> (w1159:string)
        n1256 = local read "TEST FILE NAM,E SAVED"() -> (w1152:bool)
        n1257 = call <vilib>:"Trim Whitespace.vi"("string"=w1159) -> ("trimmed string"=w1158:string)  [unwired: 1 in]
        n1258 = local read "Auto Start Test"() -> (w1162:bool)
        n1259 = String Length(string=w1158) -> (length=w1157:i32)
        n1260 = Greater?(x=w1157, y=1) -> (0:w1154:bool)
        n1261 = And(x=w1154, y=w1152) -> (x .and. y?=w1153:bool)
        n1262 = local read "RUN"() -> (w1164:bool)
        n1263 = case shown="True" w1153 {
          tunnel: [T17."Disabled" ("Disabled") T17."Enabled" ("Disabled")] -> w1155
          frame False {
          }
          frame True {
          }
        }
        n1264 = Or(x=w1164, y=w1162) -> (x .or. y?=w1163:bool)
        n1265 = property on="About" class="Bool (strict)"("DisabledEnum"=T17."Enabled" ("Disabled")) -> ()  [unwired: 2 in, 2 out]
        n1266 = case shown="False" w1163 {
          tunnel: [T17."Enabled" ("Disabled") T17."Disabled" ("Disabled")] -> w1161
          frame False {
          }
          frame True {
          }
        }
        n1267 = property on="Dashboard" class="Bool (strict)"("DisabledEnum"=w1155) -> ()  [unwired: 2 in, 2 out]
        n1268 = property on="Test Setup" class="Bool (strict)"("DisabledEnum"=T17."Disabled" ("Disabled")) -> ()  [unwired: 2 in, 2 out]
        n1269 = property on="Imaging" class="Bool (strict)"("DisabledEnum"=w1161) -> ()  [unwired: 2 in, 2 out]
        n1270 = property on="Analysis" class="Bool (strict)"("DisabledEnum"=w1161) -> ()  [unwired: 2 in, 2 out]
        n1271 = property on="Home" class="Bool (strict)"("DisabledEnum"=w1161) -> ()  [unwired: 2 in, 2 out]
        n1272 = property on="Report" class="Bool (strict)"("DisabledEnum"=w1161) -> ()  [unwired: 2 in, 2 out]
      }
    }
    n1273 = local read "Quit"() -> (w1089:bool)
    "Single" <- "Single - Graph"
  }
  n1274 = disable-structure shown="Disabled" {
    disable-tunnel: [w1441 _] -> w39
    disable-tunnel: _ -> [w1440 _]
    frame Disabled {
      n1275 = while {
        tunnel: w1440 -> [_]
        tunnel: [w1442] -> w1441
        tunnel: [w1443] -> _
        i -> [w1443]
        stop <- w1442 stop-if-true
        w1459 = u16 10 items=["1.0"=10, "1.5"=15, "2.0"=20] ("stop bits (10: 1 bit)")
        n1276 = Wait (ms)(milliseconds to wait=u32 10) -> ()  [unwired: 1 out]
        n1277 = call-poly "VISA Configure Serial Port"("VISA resource name"=refnum<visa-resource-name> "ASRL1::INSTR" ("COM PORT"), "timeout (10sec)"=u32 10, "baud rate (9600)"=u32 57600, "data bits (8)"=u16 8, "stop bits (10: 1 bit)"=w1459) -> ("VISA resource name out"=w1445:refnum<visa-resource-name>, "error out"=w1454:errorcluster)  [unwired: 9 in]
        n1278 = VISA Read(VISA resource name=w1445, byte count=u32 2 ("byte count (0)")) -> (read buffer=w1453:string)  [unwired: 1 in, 3 out]
        n1279 = String Subset(string=w1453, offset (0)=0, length (rest)=2 ("length (rest)")) -> (substring=w1452:string)
        n1280 = Match Pattern(string=w1452, regular expression="<>") -> (offset past match=w1449:i32)  [unwired: 1 in, 3 out]
        n1281 = Greater Or Equal?(x=w1449, y=0) -> (x >= y?=w1444:bool)
        n1282 = case shown="True" w1444 {
          tunnel: w1445 -> [_ w1463]
          tunnel: w1454 -> [_ w1462]
          frame False {
          }
          frame True {
            n1283 = VISA Read(VISA resource name=w1463, byte count=u32 32 ("byte count (0)"), error in (no error)=w1462) -> (read buffer=w1461:string)  [unwired: 3 out]
            n1284 = String Subset(string=w1461, offset (0)=0, length (rest)=8 ("length (rest)")) -> (substring=w1465:string)
            n1285 = String Subset(string=w1461, offset (0)=8, length (rest)=8 ("length (rest)")) -> (substring=w1466:string)
            n1286 = Decimal String To Number(string=w1466) -> (number=w1473:i32)  [unwired: 2 in, 1 out]
            n1287 = Decimal String To Number(string=w1465) -> (number=w1469:i32)  [unwired: 2 in, 1 out]
            n1288 = Divide(x=w1473, y=10000) -> ()  [unwired: 1 out]
            n1289 = Divide(x=w1469, y=1000000) -> ()  [unwired: 1 out]
          }
        }
        n1290 = local read "Quit"() -> (w1442:bool)
      }
    }
    frame Enabled {
    }
  }
  n1291 = while {
    shift-right: [w1488] -> w52
    shift-left: _ -> [w1479]
    shift-right: [w1487] -> w51
    shift-left: errorcluster {"status"=TRUE, "code"=0, "source"="Init"} ("error IO") -> [w1481]
    tunnel: [w1476] -> w42
    tunnel: [w1486] -> _
    i -> [w1486]
    stop <- w1476 stop-if-true
    n1292 = local read "Port 1a"() -> (w1482:bool)
    n1293 = local read "Port 3"() -> (w1483:bool)
    n1294 = local read "Com Port 1"() -> (w1480:refnum<visa-resource-name>)
    n1295 = Or(x=w1483, y=w1482) -> (x .or. y?=w1485:bool)
    n1296 = Unbundle(w1481) -> ("status"=→"Port 3":bool)  [unwired: 2 out]
    n1297 = Not Equal?(x=w1480, y=w1479) -> (x != y?=w1477:bool)
    n1298 = case shown="True" w1485 {
      frame False {
        w1491 = TRUE ("Visible")
        n1299 = property on="Port 1a" class="Bool (strict)"("Visible"=w1491) -> ()  [unwired: 2 in, 2 out]
        n1300 = property on="Port 3" class="Bool (strict)"("Visible"=w1491) -> ()  [unwired: 2 in, 2 out]
      }
      frame True {
        w1492 = TRUE ("Visible")
        n1301 = property on="Port 1a" class="Bool (strict)"("Visible"=w1492) -> ()  [unwired: 2 in, 2 out]
        n1302 = property on="Port 3" class="Bool (strict)"("Visible"=w1492) -> ()  [unwired: 2 in, 2 out]
      }
    }
    n1303 = Wait (ms)(milliseconds to wait=u32 40) -> ()  [unwired: 1 out]
    n1304 = case shown="True" w1477 {
      tunnel: [w1489 errorcluster {"status"=TRUE, "code"=0, "source"="Init"} ("error out")] -> w1478
      tunnel: w1481 -> [w1489 _]
      frame False {
      }
      frame True {
      }
    }
    n1305 = case shown="Error" w1478 {
      selector: w1478 -> [w1500 w1527]
      tunnel: [w1494 w1531] -> w1488
      tunnel: [w1502 w1525] -> w1487
      tunnel: w1479 -> [w1501 w1529]
      frame No Error {
        n1306 = property class="Instr"(reference=w1501, error in=w1500) -> (reference out=w1498:refnum<visa-resource-name>, error out=w1499:errorcluster, "Serial Settings:Number of Bytes at Serial Port"=w1495:u32)
        n1307 = Greater?(x=w1495, y=u32 5) -> (0:w1493:bool)
        n1308 = Not(x=w1493) -> (.not. x?=→"Port 1a":bool)
        n1309 = while {
          tunnel: [w1520] -> w1502
          tunnel: [w1519] -> w1503
          tunnel: w1499 -> [w1518]
          tunnel: w1498 -> [w1517]
          stop <- TRUE stop-if-true
          n1310 = property class="Instr" props=["Serial Settings:Number of Bytes at Serial Port"](reference=w1517, error in=w1518) -> (reference out=w1522:refnum<visa-resource-name>, error out=w1521:errorcluster)  [unwired: 1 out]
          n1311 = VISA Read(VISA resource name=w1522, byte count=u32 50, error in (no error)=w1521) -> (VISA resource name out=w1519:refnum<visa-resource-name>, read buffer=w1504:string, error out=w1520:errorcluster)  [unwired: 1 out]
          "UNI READ" <- w1504
          n1312 = Spreadsheet String To Array(delimiter (Tab)=";", format string="", spreadsheet string=w1504, array type (2D Dbl)=dbl[] []) -> (array=w1514:dbl[])
          n1313 = Index Array(array=w1514) -> (element #1=→"LVDT MIN":dbl, element #2=→"LVDT MAX":dbl, element #3=→"LVDT Peak":dbl, element #4=→"pizo raw":dbl, element #5=→"Friction":dbl, element #6=→"cof 2":dbl)  [unwired: 6 in]
        }
        n1314 = VISA Flush I/O Buffer(VISA resource name=w1503) -> (VISA resource name out=w1494:refnum<visa-resource-name>)  [unwired: 2 in, 1 out]
      }
      frame Error {
        w1537 = u16 0 items=["None", "XON/XOFF", "RTS/CTS", "XON/XOFF & RTS/CTS", "DTR/DSR", "XON/XOFF & DTR/DSR"] ("flow control (0:none)  2")
        w1535 = u16 10 items=["1.0"=10, "1.5"=15, "2.0"=20] ("stop bits 2")
        w1533 = u16 0 items=["None", "Odd", "Even", "Mark", "Space"] ("parity 2")
        w1534 = u32 10000  # timeout (10sec)
        n1315 = VISA Close(VISA resource name=w1529, error in (no error)=w1527) -> (error out=w1530:errorcluster)
        n1316 = local write "Port 1a"(FALSE ("Port 1a")) -> ()
        n1317 = local read "Com Port 1"() -> (w1524:refnum<visa-resource-name>)
        n1318 = call <vilib>:"Clear Errors.vi"("error in (no error)"=w1530) -> ("error out"=w1528:errorcluster)  [unwired: 5 in, 1 out]
        n1319 = call-poly "VISA Configure Serial Port"("VISA resource name"=w1524, "timeout (10sec)"=w1534, "baud rate (9600)"=u32 250000 ("baud rate  2"), "data bits (8)"=u16 8 ("data bits  2"), "parity (0:none)"=w1533, "error in (no error)"=w1528, "stop bits (10: 1 bit)"=w1535, "flow control (0:none)"=w1537) -> ("VISA resource name out"=w1538:refnum<visa-resource-name>, "error out"=w1539:errorcluster)  [unwired: 6 in]
        n1320 = flat-sequence {
          tunnel: w1538 -> [w1541]
          tunnel: w1539 -> [w1540]
          tunnel: [w1541] -> w1531
          tunnel: [w1540] -> w1525
          frame #0 {
            n1321 = Wait (ms)(milliseconds to wait=u32 50) -> ()  [unwired: 1 out]
          }
        }
        "Residual Uno" <- ""
        "Port 1 Error" <- w1525
      }
    }
    n1322 = local read "Quit"() -> (w1476:bool)
    "Error Uno" <- w1481
  }
  n1323 = while {
    stop <- w1551 stop-if-true
    # "V0OLTAGE TO STROKE (peice vise calibration)"
    n1324 = Wait (ms)(milliseconds to wait=u32 10) -> ()  [unwired: 1 out]
    n1325 = local read "LVDT Peak"() -> (w1548:dbl)
    n1326 = formula code="// Dynamic Parameterized Linear Interpolation Node\n// Inputs: vpp_val, voltages (Array), distances (Array)\n// Outputs: stroke\n\nint i = 0;\nint segments = 11; // 12 points make 11 interpolation segments\n\n// 1. Lower Boundary Clamp\nif (vpp_val <= voltages[0]) {\n    stroke = distances[0];\n}\n// 2. Upper Boundary Clamp\nelse if (vpp_val >= voltages[segments]) {\n    stroke = distances[segments];\n}\n// 3. Dynamic Segment Search Loop\nelse {\n    stroke = distances[0]; // Fallback baseline\n    for (i = 0; i < segments; i++) {\n        if (vpp_val >= voltages[i] && vpp_val <= voltages[i+1]) {\n            // Standard linear interpolation formula using array lookups\n            stroke = distances[i] + (vpp_val - voltages[i]) * (distances[i+1] - distances[i]) / (voltages[i+1] - voltages[i]);\n            break; // Segment found, safely exit the loop\n        }\n    }\n}"("vpp_val"=w1548, "voltages"="calibration values", "distances"="STROKE") -> ("stroke"=w1545:dbl)
    "LVDT STROKE" <- w1545
    n1327 = local read "Calibration Tare Value"() -> (w1546:dbl)
    n1328 = local read "Calibration Tare"() -> (w1544:bool)
    n1329 = local read "Quit"() -> (w1551:bool)
    n1330 = Subtract(x=w1545, y=w1546) -> (x-y=→"LVDT STROKE  Calibration":dbl)
    n1331 = case shown="True" w1544 {
      selector: w1544 -> [_ w1553]
      tunnel: w1545 -> [_ w1554]
      frame False {
      }
      frame True {
        n1332 = Not(x=w1553) -> (.not. x?=w1552:bool)
        n1333 = local write "Calibration Tare"(w1552) -> ()
        "Calibration Tare Value" <- w1554
      }
    }
  }
  n1334 = while {
    stop <- w1574 stop-if-true
    n1335 = call <vilib>:"High Resolution Polling Wait.vi"("seconds to wait"=0.02) -> ()  [unwired: 10 in, 1 out]
    n1336 = local read "Due read"() -> (w1572:string)
    n1337 = Spreadsheet String To Array(delimiter (Tab)=";", format string="", spreadsheet string=w1572, array type (2D Dbl)=string[] []) -> (array=w1569:string[])
    n1338 = Fract/Exp String To Number(string=w1569) -> (number=w1568:dbl[])  [unwired: 3 in, 1 out]
    n1339 = Index Array(array=w1568) -> (element #1=→"Sample Temperature":dbl, element #2=→"Target Sample Temperature":dbl, element #3=→"Current Duty Cycle":dbl, element #4=→"Ambient Temperature":dbl, element #5=→"Dac Status":dbl, element #6=→"Vpp":dbl, element #7=→"Active Error Code":dbl, element #8=→"Kp":dbl, element #9=→"Ki":dbl, element #10=→"Kd":dbl, element #11=→"SampleRaw":dbl, element #12=→"AmbRaw":dbl)  [unwired: 12 in]
    n1340 = local read "Quit"() -> (w1574:bool)
  }
  n1341 = while {
    shift-right: [w1588] -> w37
    shift-left: _ -> [w1579]
    shift-right: [w1587] -> w36
    shift-left: errorcluster {"status"=FALSE, "code"=0, "source"="Init"} ("error out") -> [w1581]
    tunnel: [w1576] -> w41
    tunnel: [w1586] -> _
    i -> [w1586]
    stop <- w1576 stop-if-true
    n1342 = local read "Com Port 2"() -> (w1580:refnum<visa-resource-name>)
    n1343 = local read "Port 2a"() -> (w1582:bool)
    n1344 = Unbundle(w1581) -> ("status"=→"Port 4":bool)  [unwired: 2 out]
    n1345 = call <vilib>:"High Resolution Polling Wait.vi"("seconds to wait"=0.02) -> ()  [unwired: 10 in, 1 out]
    n1346 = local read "Port 4"() -> (w1583:bool)
    n1347 = Not Equal?(x=w1580, y=w1579) -> (x != y?=w1578:bool)
    n1348 = Or(x=w1583, y=w1582) -> (x .or. y?=w1585:bool)
    n1349 = case shown="False" w1585 {
      frame False {
        w1591 = TRUE ("Visible")
        n1350 = property on="Port 2a" class="Bool (strict)"("Visible"=w1591) -> ()  [unwired: 2 in, 2 out]
        n1351 = property on="Port 4" class="Bool (strict)"("Visible"=w1591) -> ()  [unwired: 2 in, 2 out]
      }
      frame True {
        w1592 = TRUE ("Visible")
        n1352 = property on="Port 2a" class="Bool (strict)"("Visible"=w1592) -> ()  [unwired: 2 in, 2 out]
        n1353 = property on="Port 4" class="Bool (strict)"("Visible"=w1592) -> ()  [unwired: 2 in, 2 out]
      }
    }
    n1354 = case shown="True" w1578 {
      tunnel: [w1589 errorcluster {"status"=TRUE, "code"=0, "source"="Init"} ("error out")] -> w1577
      tunnel: w1581 -> [w1589 _]
      frame False {
      }
      frame True {
      }
    }
    n1355 = case shown="No Error" w1577 {
      selector: w1577 -> [w1603 w1634]
      tunnel: [w1596 w1639] -> w1588
      tunnel: [w1604 w1632] -> w1587
      tunnel: w1579 -> [w1606 w1637]
      frame No Error {
        n1356 = property class="Instr" props=["Serial Settings:Number of Bytes at Serial Port"](reference=w1606, error in=w1603) -> (reference out=w1597:refnum<visa-resource-name>, error out=w1602:errorcluster)  [unwired: 1 out]
        n1357 = while {
          tunnel: [w1614] -> w1598
          tunnel: [w1613] -> w1599
          tunnel: w1602 -> [w1612]
          tunnel: w1597 -> [w1611]
          tunnel: [w1610] -> _
          i -> [w1610]
          stop <- TRUE stop-if-true
          n1358 = property class="Instr" props=["Serial Settings:Number of Bytes at Serial Port"](reference=w1611, error in=w1612) -> (reference out=w1616:refnum<visa-resource-name>, error out=w1615:errorcluster)  [unwired: 1 out]
          n1359 = VISA Read(VISA resource name=w1616, byte count=u32 1000, error in (no error)=w1615) -> (VISA resource name out=w1613:refnum<visa-resource-name>, read buffer=→"Due read":string, error out=w1614:errorcluster)  [unwired: 1 out]
        }
        n1360 = local read "Command"() -> (w1594:string)
        n1361 = call <vilib>:"Trim Whitespace.vi"("string"=w1594) -> ("trimmed string"=w1593:string)  [unwired: 1 in]
        n1362 = Not Equal?(x=w1593, y="") -> (x != y?=w1600:bool)
        n1363 = case shown="True" w1600 {
          tunnel: w1599 -> [w1618 w1623]
          tunnel: [w1618 w1627] -> w1605
          tunnel: w1598 -> [w1617 w1622]
          tunnel: [w1617 w1625] -> w1604
          tunnel: w1593 -> [_ w1621]
          tunnel: [_ w1624] -> _
          frame False {
            # "DATA  WRITE LOOP"
          }
          frame True {
            n1364 = Concatenate Strings(w1621, "\r\n") -> (w1620:string)
            n1365 = VISA Write(VISA resource name=w1623, write buffer=w1620, error in (no error)=w1622) -> (VISA resource name out=w1627:refnum<visa-resource-name>, return count=w1624:u32, error out=w1626:errorcluster)
            n1366 = flat-sequence {
              tunnel: w1626 -> [w1629]
              tunnel: [w1629] -> w1625
              frame #0 {
                n1367 = local write "Command"("" ("Command")) -> ()
                n1368 = Wait (ms)(milliseconds to wait=u32 5) -> ()  [unwired: 1 out]
              }
            }
          }
        }
        n1369 = VISA Flush I/O Buffer(VISA resource name=w1605) -> (VISA resource name out=w1596:refnum<visa-resource-name>, error out=→"error out 9":errorcluster)  [unwired: 2 in]
      }
      frame Error {
        w1645 = u16 0 items=["None", "XON/XOFF", "RTS/CTS", "XON/XOFF & RTS/CTS", "DTR/DSR", "XON/XOFF & DTR/DSR"] ("flow control (0:none)  2")
        w1643 = u16 10 items=["1.0"=10, "1.5"=15, "2.0"=20] ("stop bits 2")
        w1641 = u16 0 items=["None", "Odd", "Even", "Mark", "Space"] ("parity 2")
        w1642 = u32 10000  # timeout (10sec)
        n1370 = VISA Clear(VISA resource name=w1637, error in (no error)=w1634) -> (VISA resource name out=w1636:refnum<visa-resource-name>, error out=w1635:errorcluster)
        n1371 = VISA Close(VISA resource name=w1636, error in (no error)=w1635) -> (error out=w1638:errorcluster)
        n1372 = call <vilib>:"Clear Errors.vi"("error in (no error)"=w1638) -> ()  [unwired: 5 in, 2 out]
        n1373 = local read "Com Port 2"() -> (w1631:refnum<visa-resource-name>)
        "visa due" <- w1631
        n1374 = call-poly "VISA Configure Serial Port"("VISA resource name"=w1631, "timeout (10sec)"=w1642, "baud rate (9600)"=u32 250000 ("baud rate  2"), "data bits (8)"=u16 8 ("data bits  2"), "parity (0:none)"=w1641, "stop bits (10: 1 bit)"=w1643, "flow control (0:none)"=w1645) -> ("VISA resource name out"=w1646:refnum<visa-resource-name>, "error out"=w1647:errorcluster)  [unwired: 7 in]
        n1375 = flat-sequence {
          tunnel: w1646 -> [w1649]
          tunnel: w1647 -> [w1648]
          tunnel: [w1649] -> w1639
          tunnel: [w1648] -> w1632
          frame #0 {
            n1376 = Wait (ms)(milliseconds to wait=u32 50) -> ()  [unwired: 1 out]
          }
        }
        "Residual Due" <- ""
        "Port 2 Error" <- w1632
      }
    }
    n1377 = local read "Quit"() -> (w1576:bool)
    "Error Due" <- w1581
  }
  n1378 = local write "FRICVALZ"(0.0 ("FRICVALZ")) -> ()
  n1379 = property on="RUN" class="Bool (strict)"("Visible"=TRUE) -> ()  [unwired: 2 in, 2 out]
  n1380 = while {
    tunnel: [w1666] -> _
    tunnel: [w1651] -> w54
    i -> [w1666]
    stop <- w1651 stop-if-true
    n1381 = local read "conststatus"() -> (w1655:dbl)
    n1382 = local read "Main Tab"() -> (w1653:T2)
    n1383 = local read "EDIT"() -> (w1672:bool)
    n1384 = local read "Rate"() -> (w1671:dbl)
    n1385 = case shown="True" w1672 {
      tunnel: [FALSE TRUE] -> w1658
      frame False {
      }
      frame True {
      }
    }
    n1386 = property on="Time slide" class="Slide (strict)"("Scale.Range:Maximum"=2500.0) -> ()  [unwired: 2 in, 2 out]
    n1387 = Equal?(x=w1653, y=T26."About" ("Main Tab")) -> (x = y?=w1664:bool)
    n1388 = Equal?(x=w1655, y=0.0) -> (x = y?=w1656:bool)
    n1389 = Divide(x=1.0, y=w1671) -> (x/y=w1667:dbl)
    "Time 2" <- w1667
    n1390 = case shown="True" w1656 {
      frame False {
      }
      frame True {
        # "C:\\WinDucom\\calibrate WO 2391.dcf"
        n1391 = local write "Lan flag"(22) -> ()
        n1392 = local write "conststatus"(10.0 ("rpm value : 2")) -> ()
        n1393 = String To Path(string="C:\\LAB-IQ\\calibrate WO 2465.dcf") -> (path=w1678:path)
        n1394 = Open/Create/Replace File "Open File"(file path (use dialog)=w1678) -> (refnum out=w1676:refnum<file>)  [unwired: 5 in, 2 out]
        n1395 = for {
          N: 23 -> [_]
          tunnel: w1676 -> [w1687]
          i -> [w1681]
          (unwired) TRUE ("line mode (F)")
          n1396 = Read from Text File "Read File"(file (use dialog)=w1687) -> (text=w1686:string)  [unwired: 3 in, 3 out]
          n1397 = Match Pattern(string=w1686, regular expression="]") -> (after substring=w1684:string)  [unwired: 1 in, 3 out]
          n1398 = String Subset(string=w1686, offset (0)=5, length (rest)=10 ("length (rest)")) -> (substring=w1679:string)
          n1399 = Fract/Exp String To Number(string=w1679) -> (number=w1680:dbl)  [unwired: 3 in, 1 out]
          n1400 = Match Pattern(string=w1684, regular expression="-") -> (before substring=w1682:string)  [unwired: 1 in, 3 out]
          n1401 = case shown="19" w1681 {
            tunnel: w1680 -> [w1690 w1691 w1692 w1693 _ _ _ w1698 w1699 _ w1700 w1701 w1702 w1703 w1704 w1705 _ w1706 w1707 _ _ _ _ _]
            tunnel: w1682 -> [_ _ _ _ w1694 w1695 w1696 _ _ _ _ _ _ _ _ _ _ _ _ w1708 w1709 w1710 w1711 _]
            frame 0 {
              n1402 = local write "FRIC. FORCE :"(w1690) -> ()
            }
            frame 1 {
              n1403 = local write "TEMPERATURE :"(w1691) -> ()
            }
            frame 2 {
              n1404 = local write "HUMIDITY:"(w1692) -> ()
            }
            frame 3 {
              n1405 = local write "AIR TEMPERATURE :"(w1693) -> ()
            }
            frame 4 {
              n1406 = local write "Com Port 1"(w1694) -> ()
            }
            frame 5 {
              n1407 = local write "Com Port 2"(w1695) -> ()
              n1408 = local write "visa due"(w1695) -> ()
            }
            frame 6 {
              n1409 = String To Path(string=w1696) -> (path=w1697:path)
              n1410 = local write "File Path"(w1697) -> ()
              "String" <- w1696
            }
            frame 7 {
              n1411 = local write "DISPLACEMENT :"(w1698) -> ()
            }
            frame 8 {
              n1412 = local write "STROKE GAIN :"(w1699) -> ()
            }
            frame 9 {
            }
            frame 10 {
              n1413 = local write "Language Selection"(w1700) -> ()
            }
            frame 11 {
              n1414 = local write "CH-POWER +"(w1701) -> ()
            }
            frame 12 {
              n1415 = local write "CH-POWER -"(w1702) -> ()
            }
            frame 13 {
              n1416 = local write "CH-HEATER"(w1703) -> ()
            }
            frame 14 {
              n1417 = local write "CH-HUMIDITY WET"(w1704) -> ()
            }
            frame 15 {
              n1418 = local write "CH-HUMIDITY DRY"(w1705) -> ()
            }
            frame 16 {
            }
            frame 17 {
              n1419 = local write "AIR TEMP INTERCEPT:"(w1706) -> ()
            }
            frame 18 {
              n1420 = local write "TEMP INTERCEPT:"(w1707) -> ()
            }
            frame 21 {
              n1421 = local write "S.NO"(w1708) -> ()
            }
            frame 22 {
              n1422 = local write "Com Port 3"(w1709) -> ()
            }
            frame 20 {
              n1423 = local write "Camera Port :"(w1710) -> ()
            }
            frame 19 {
              n1424 = local write "C3 :"(w1711) -> ()
            }
            frame 23, Default {
            }
          }
        }
      }
    }
    n1425 = Select(t=u32 2500 ("milliseconds to wait"), s=w1664, f=u32 500 ("milliseconds to wait")) -> (s? t:f=w1662:u32)
    n1426 = Multiply(x=w1667, y=w1662) -> (x*y=w1669:dbl)
    n1427 = property on="Time slide" class="Slide (strict)"("Visible"=w1658) -> ()  [unwired: 2 in, 2 out]
    n1428 = call "Elapsed Time2"("Time Target (s)"=w1669, "Auto Reset"=TRUE) -> ("Time has Elapsed"=w1659:bool)  [unwired: 10 in, 7 out]
    n1429 = case shown="True" w1659 {
      frame False {
      }
      frame True {
        n1430 = stacked-sequence {
          frame #0 {
            # "DATA PROCESSING"
            # "115 mV/N"
            n1431 = local read "Sample Temperature"() -> (w1712:dbl)
            "TEMP 2" <- w1712
            "TEMP 3" <- w1712
            n1432 = local read "RH Numeric:"() -> (w1719:dbl)
            n1433 = local read "HUMIDITY:"() -> (w1720:dbl)
            n1434 = local read "FRICVALZ"() -> (w1731:dbl)
            n1435 = local read "Friction"() -> (w1715:dbl)
            n1436 = local write "TEMP"(w1712) -> ()
            n1437 = Multiply(x=w1719, y=w1720) -> (x*y=→"Humidity ( %RH )" →"Hum" →"Hum 2":dbl)
            n1438 = Subtract(x=w1715, y=w1731) -> (x-y=w1726:dbl)
            "FF 2" <- w1726
            "FF 4" <- w1726
            n1439 = local read "Ambient Temperature"() -> (→"AIR TEMP":dbl)
            n1440 = local read "TEMP"() -> (w1730:dbl)
            n1441 = local write "FF 3"(w1726) -> ()
            n1442 = Compound Arithmetic op=OR("FRICVALZ 4", "FRICVALZ 3", "FRICVALZ 2") -> (w1722:bool)
            n1443 = case shown="True" w1722 {
              tunnel: w1715 -> [_ w1737]
              frame False {
              }
              frame True {
                w1736 = FALSE ("FRICVALZ")
                n1444 = local write "FRICVALZ 3"(w1736) -> ()
                n1445 = local write "FRICVALZ 2"(w1736) -> ()
                n1446 = local write "FRICVALZ 4"(w1736) -> ()
                "FRICVALZ" <- w1737
              }
            }
            n1447 = Not A Number/Path/Refnum?(number/path/refnum=w1730) -> (NaN/Path/Refnum?=w1729:bool)
            n1448 = Not A Number/Path/Refnum?(number/path/refnum=w1726) -> (NaN/Path/Refnum?=w1728:bool)
            n1449 = Divide(x=w1726, y=1.96) -> (x/y=w1723:dbl)
            n1450 = Compound Arithmetic op=OR(w1729, w1728) -> (w1727:bool)
            n1451 = Not A Number/Path/Refnum?(number/path/refnum=w1723) -> (NaN/Path/Refnum?=w1724:bool)
            n1452 = case shown="True" w1727 {
              frame False {
              }
              frame True {
                n1453 = local write "TEMP"(0.0 ("TEMP")) -> ()
                n1454 = local write "FF 2"(0.0 ("FF 2")) -> ()
                n1455 = local write "reinit"(TRUE ("reinit")) -> ()
              }
            }
            n1456 = Select(t=0.0, s=w1724, f=w1723) -> (s? t:f=w1714:dbl)
            "COF 2" <- w1714
            n1457 = local write "COF 3"(w1714) -> ()
          }
        }
      }
    }
    n1458 = Wait (ms)(milliseconds to wait=u32 50) -> ()  [unwired: 1 out]
    n1459 = local read "Quit"() -> (w1651:bool)
    "Rate" <- 2500.0 ("No of Samples")
  }
  n1460 = while {
    tunnel: w57 -> [_]
    tunnel: [w1764] -> _
    tunnel: [w1740] -> w56
    i -> [w1764]
    stop <- w1740 stop-if-true
    # "C:\\LAB-IQ-NXT\\Scar View.exe"
    n1461 = local read "OK Button 16"() -> (w1753:bool)
    n1462 = local read "Main Tab"() -> (w1746:T2)
    n1463 = local read "service 3"() -> (w1747:bool)
    n1464 = local read "OPEN 6"() -> (w1749:bool)
    n1465 = local read "EDIT 2"() -> (w1751:bool)
    n1466 = flat-sequence {
      frame #0 {
        n1467 = local read "SAVE 2"() -> (w2366:bool)
        n1468 = stacked-sequence {
          frame #0 {
            n1469 = local read "EDIT"() -> (w2420:bool)
            n1470 = case shown="True" w2420 {
              tunnel: [u8 2 ("Disabled") u8 0 ("Disabled")] -> _
              frame False {
                w2422 = FALSE
                n1471 = local write "Password"("") -> ()
                n1472 = property on="SrvM CP" class="Bool (strict)"("Visible"=w2422) -> ()  [unwired: 2 in, 2 out]
                n1473 = property on="message" class="Str"("Visible"=w2422) -> ()  [unwired: 2 in, 2 out]
                n1474 = local write "x = y?"(w2422) -> ()
                n1475 = property on="Password" class="Str"("Visible"=w2422) -> ()  [unwired: 2 in, 2 out]
                n1476 = property on="ENTER THE NEW PASSWORD" class="Str"("Visible"=w2422) -> ()  [unwired: 2 in, 2 out]
                n1477 = property on="ENTER CURRENT PASSWORD" class="Str"("Visible"=w2422) -> ()  [unwired: 2 in, 2 out]
                n1478 = local write "SrvM CP"(w2422) -> ()
              }
              frame True {
                w2425 = TRUE
                n1479 = property on="SrvM CP" class="Bool (strict)"("Visible"=w2425) -> ()  [unwired: 2 in, 2 out]
                n1480 = property on="Password" class="Str"("Visible"=w2425) -> ()  [unwired: 2 in, 2 out]
              }
            }
            "dipl pwd" <- "@143$\n" ("dipl pwd")
          }
          frame #1 {
            # "Gain password"
            n1481 = String To Byte Array(string="ENTER CURRENT PASSWORD") -> (unsigned byte array=w2430:u8[])
            n1482 = Search 1D Array(1D array=w2430, element=u8 10) -> (index of element=w2433:i32)  [unwired: 1 in]
            n1483 = Index Array(array=w2430, index=w2433) -> (element=w2429:u8)
